vi "test Parse Section Identifier.vi"(11 "Test Case In":refnum<class "test EDS.lvclass">) -> (0 "error out":errorcluster, 3 "Test Case Out":refnum<class "test EDS.lvclass">)   [LabVIEW 2024, in "test EDS.lvclass"]
uses:
  test EDS.lvclass
  C:/Program Files/National Instruments/LabVIEW 2024/vi.lib/Astemes/LUnit/Test Case.lvclass
  <vilib>/Astemes/LUnit/Test Case.lvclass/Test Case.ctl
  <vilib>/Astemes/LUnit/Append Fail Result.vi
  <vilib>/Astemes/LUnit/Append Pass Result.vi
  <vilib>/Astemes/LUnit/Run In UI.vi
  <vilib>/Utility/error.llb/Clear Errors.vi
  <vilib>/Astemes/LUnit/Test Case.lvclass
  Core/Section Name/Section Name.lvclass
panel:
  out "appended array":string[][](array[string])
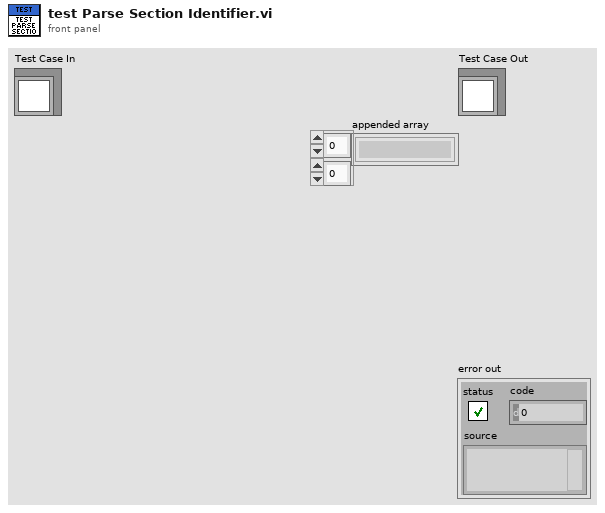
[diagram p1: front panel]
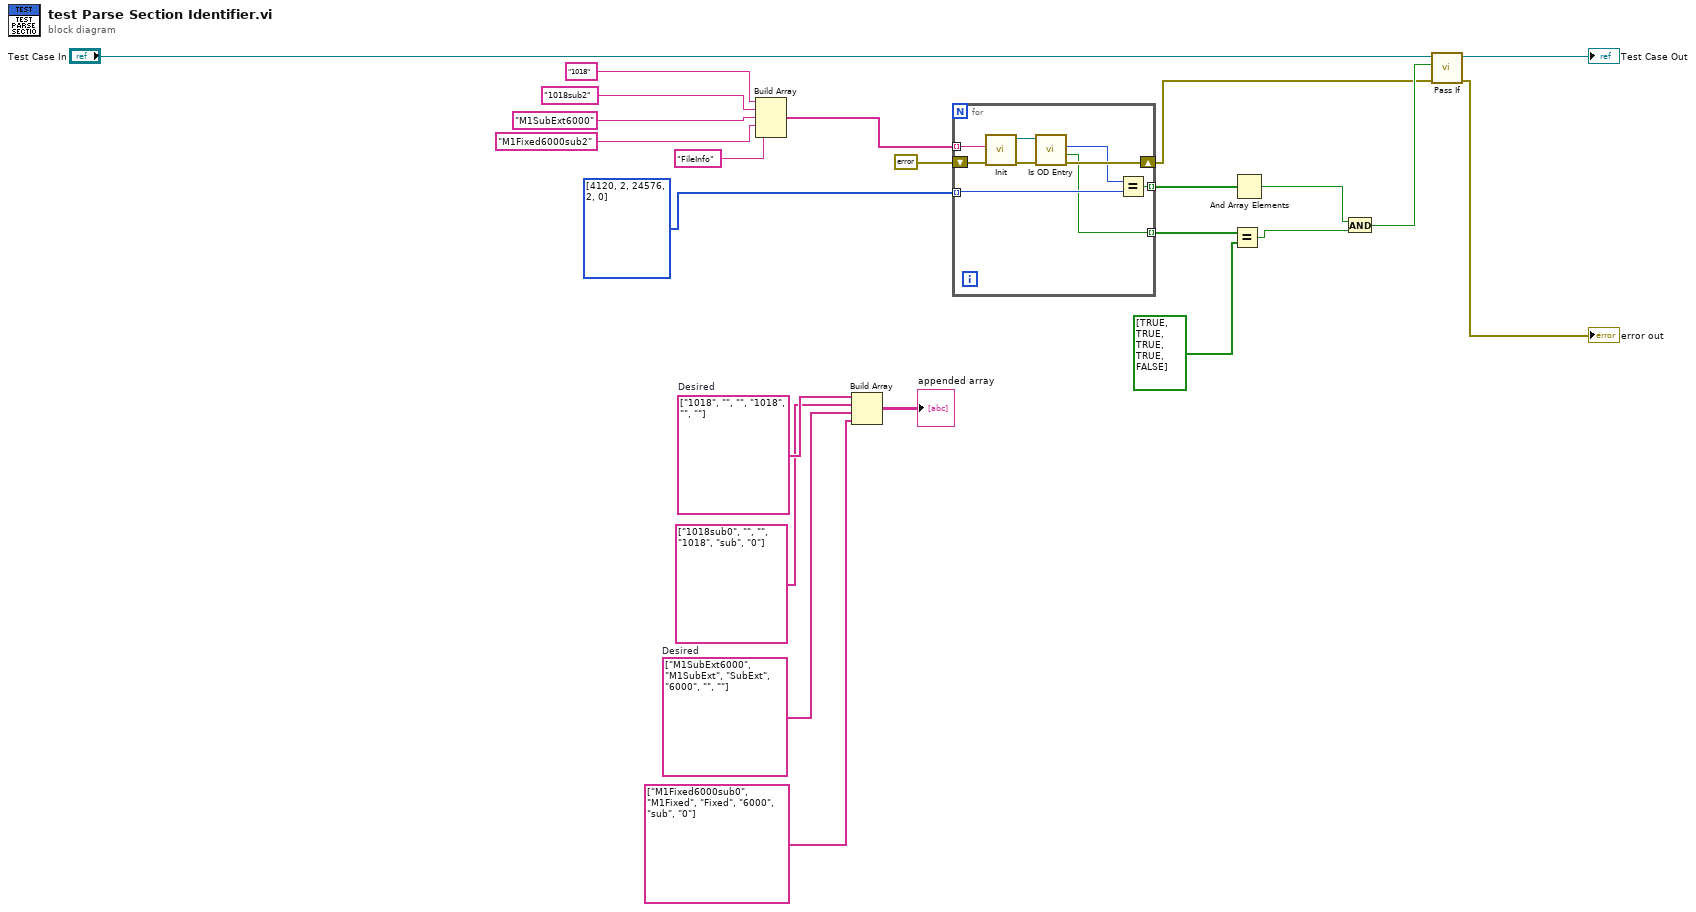
[diagram p0: block diagram]
diagram:
  w16 = string[] ["1018", "", "", "1018", "", ""]  # Desired
  w14 = string[] ["M1SubExt6000", "M1SubExt", "SubExt", "6000", "", ""]  # Desired
  n1 = Build Array("1018", "1018sub2", "M1SubExt6000", "M1Fixed6000sub2", "FileInfo" ("element")) -> (w2:string[])
  n2 = Build Array(w16, string[] ["1018sub0", "", "", "1018", "sub", "0"] ("Desired"), w14, string[] ["M1Fixed6000sub0", "M1Fixed", "Fixed", "6000", "sub", "0"] ("Desired")) -> (→"appended array":string[][])
  n3 = for {
    shift-right: [w32] -> w8
    shift-left: errorcluster {"status"=FALSE, "code"=0, "source"=""} ("Error Out") -> [w25]
    tunnel: [w28] -> w5 mode=indexing
    tunnel: u16[] [4120, 2, 24576, 2, 0] ("Array") -> [w31] mode=indexing
    tunnel: [w30] -> w11 mode=indexing
    tunnel: w2 -> [w27] mode=indexing
    n4 = call "Init.vi"("error in"=w25, "Section Name"=w27) -> ("error out"=w24:errorcluster, "Section Name out"=w26:refnum<class "Section Name.lvclass">)  [unwired: 8 in]
    n5 = call "Is OD Entry.vi"("error in"=w24, "Section Name in"=w26) -> ("error out"=w32:errorcluster, "Is OD Entry?"=w28:bool, "Index"=w29:u16)  [unwired: 6 in, 1 out]
    n6 = Equal?(x=w29, y=w31) -> (x = y?=w30:bool)
  }
  n7 = Equal?(x=w5, y=bool[] [TRUE, TRUE, TRUE, TRUE, FALSE]) -> (x = y?=w3:bool)
  n8 = And Array Elements(Boolean array=w11) -> (logical AND=w9:bool)
  n9 = And(x=w9, y=w3) -> (x .and. y?=w10:bool)
  n10 = call <vilib>:"Pass If.vi"("error in (no error)"=w8, "Pass?"=w10, "LUnit Test Case In"="Test Case In") -> ("error out"=→"error out":errorcluster, "LUnit Test Case Out"=→"Test Case Out":refnum<class "test EDS.lvclass">)  [unwired: 7 in]
